vi "WF_Collector.vi"(8 "error in (no error)":errorcluster, 10 "LoopCounter":i32, 11 "waveform data ClusterIn":waveform(dbl)[](array[waveform])) -> (0 "error out":errorcluster, 3 "waveform data ClusterOut":waveform(dbl)[](array[waveform]))   [LabVIEW 2018]
uses:
  <vilib>/Waveform/WDTOps.llb/WDT Append Waveforms DBL.vi
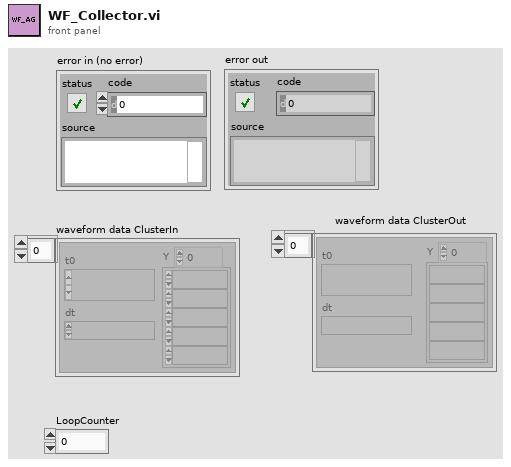
[diagram p1: front panel]
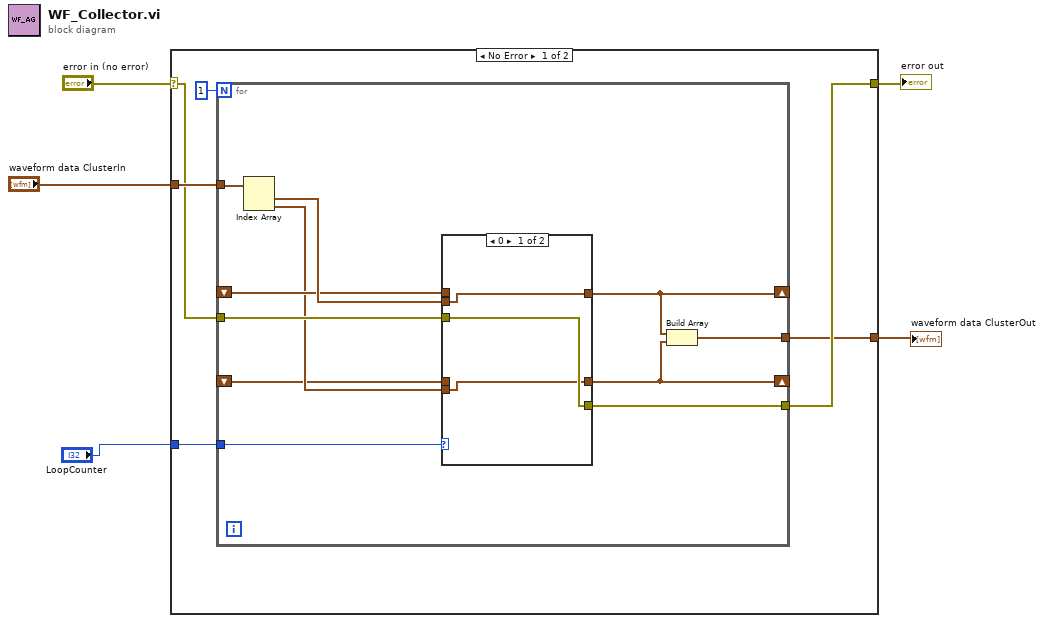
[diagram p0: block diagram]
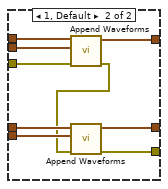
[diagram p2: hidden frame]
diagram:
  n1 = case shown="No Error" "error in (no error)" {
    selector: "error in (no error)" -> [w9 w35]
    tunnel: [w8 w35] -> w4
    tunnel: "waveform data ClusterIn" -> [w10 _]
    tunnel: "LoopCounter" -> [w7 _]
    tunnel: [w6 _] -> w1
    frame No Error {
      n2 = for {
        N: 1 -> [_]
        tunnel: w10 -> [w22]
        shift-right: [w14] -> _
        shift-left: _ -> [w20]
        tunnel: w9 -> [w19]
        shift-right: [w13] -> _
        shift-left: _ -> [w17]
        tunnel: [w16] -> w8
        tunnel: w7 -> [w15]
        tunnel: [w12] -> w6
        n3 = Index Array(array=w22) -> (element #1=w21:waveform(dbl), element #2=w18:waveform(dbl))  [unwired: 2 in]
        n4 = case shown="0" w15 {
          tunnel: w21 -> [w24 w34]
          tunnel: [w24 w33] -> w14
          tunnel: w20 -> [_ w32]
          tunnel: w19 -> [w25 w31]
          tunnel: w18 -> [w23 w30]
          tunnel: [w23 w29] -> w13
          tunnel: w17 -> [_ w28]
          tunnel: [w25 w26] -> w16
          frame 0 {
          }
          frame 1, Default {
            n5 = call-poly <vilib>:"Append Waveforms.vi"("error in (no error)"=w31, "waveform B"=w34, "waveform A"=w32) -> ("error out"=w27:errorcluster, "waveform out"=w33:waveform(dbl))  [unwired: 7 in]
            n6 = call-poly <vilib>:"Append Waveforms.vi"("error in (no error)"=w27, "waveform B"=w30, "waveform A"=w28) -> ("error out"=w26:errorcluster, "waveform out"=w29:waveform(dbl))  [unwired: 7 in]
          }
        }
        n7 = Build Array(w14, w13) -> (w12:waveform(dbl)[])
      }
    }
    frame Error {
    }
  }
  "error out" <- w4
  "waveform data ClusterOut" <- w1
